vi "Load Default Measurements.vi"(8 "error in (no error)":errorcluster, 11 "Measurement Interface in":refnum<class "Measurement Interface.lvclass">) -> (0 "error out":errorcluster, 3 "Measurement Interface out":refnum<class "Measurement Interface.lvclass">)   [LabVIEW 2016, in "Measurement Interface.lvlib" / "Measurement Interface.lvclass"]
uses:
  Measurement Interface.lvclass
  Measurement Interface.lvclass/Measurement Interface.ctl
  Plugins/TestStand API Tools (TSAT).lvlibp/Sequence File Actions/TSAT Sequence File Actions.lvlib
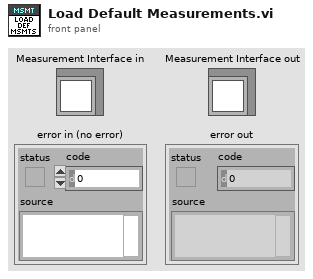
[diagram p1: front panel]
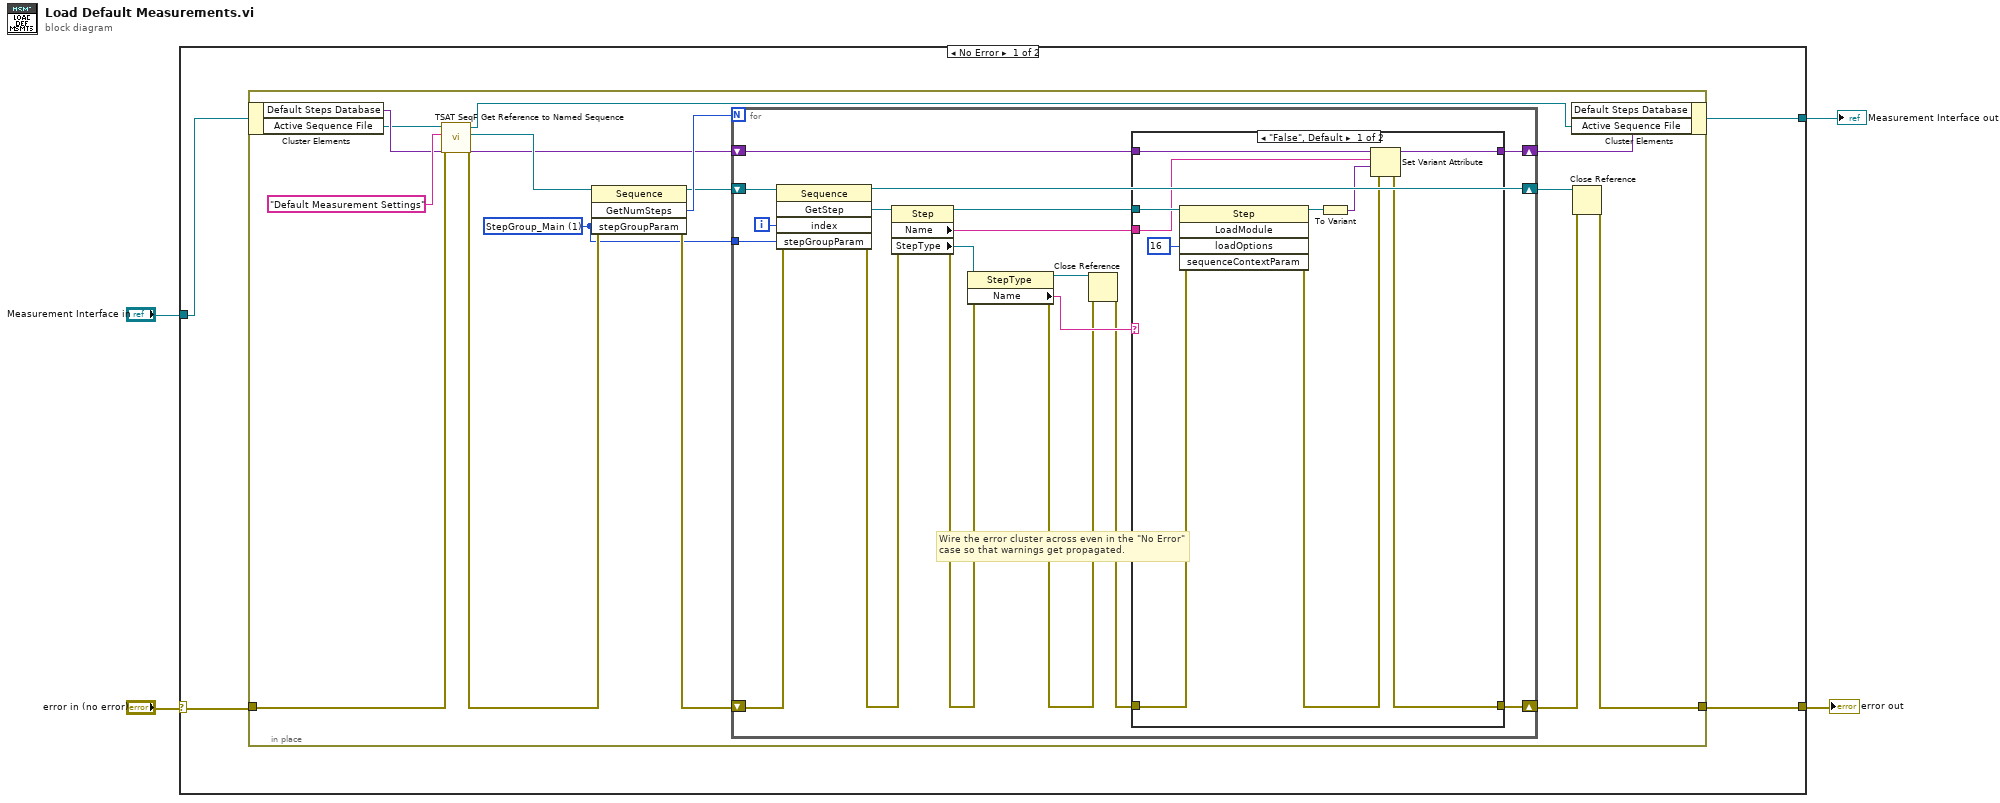
[diagram p0: block diagram]
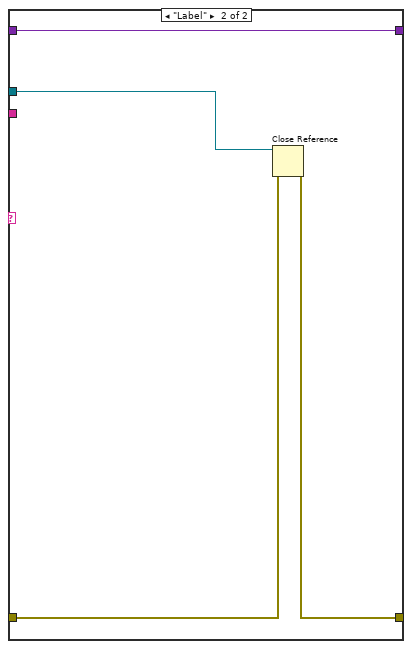
[diagram p2: hidden frame]
diagram:
  n1 = case shown="No Error" "error in (no error)" {
    selector: "error in (no error)" -> [w8 w57]
    tunnel: [w5 w57] -> w3
    tunnel: [w6 w56] -> w1
    tunnel: "Measurement Interface in" -> [w7 w56]
    frame No Error {
      # "Wire the error cluster across even in the \"No Error\"\ncase so that warnings get propagated."
      n2 = in-place {
        in-place-border: w8 -> [w23]
        in-place-border: [w11] -> w5
        w16 = 1 items=["StepGroup_Setup", "StepGroup_Main", "StepGroup_Cleanup"] ("stepGroupParam")
        n3 = in-place-cluster #1(w7) -> ("Default Steps Database"=w15:variant, "Active Sequence File"=w10:refnum<k7>)
        n4 = call "TSAT SeqF Get Reference to Named Sequence.vi"("Error In"=w23, "Seqeunce to Retrieve"="Default Measurement Settings", "Sequence File In"=w10) -> ("Error Out"=w20:errorcluster, "Named Sequence"=w21:refnum<k7>, "Sequence File Out"=w9:refnum<k7>)  [unwired: 6 in]
        n5 = invoke class="Sequence" method="GetNumSteps"(reference=w21, error in=w20, "stepGroupParam"=w16) -> (reference out=w18:refnum<k7>, error out=w17:errorcluster, "GetNumSteps"=w19:i32)  [unwired: 1 in, 1 out]
        n6 = for {
          N: w19 -> [_]
          shift-right: [w35] -> w13
          shift-left: w18 -> [w41]
          shift-right: [w29] -> w12
          shift-left: w17 -> [w39]
          tunnel: w16 -> [w38]
          shift-right: [w24] -> w14
          shift-left: w15 -> [w25]
          i -> [w40]
          n7 = invoke class="Sequence" method="GetStep"(reference=w41, error in=w39, "index"=w40, "stepGroupParam"=w38) -> (reference out=w35:refnum<k7>, error out=w36:errorcluster, "GetStep"=w37:refnum<k7>)  [unwired: 1 in, 2 out]
          n8 = property class="Step"(reference=w37, error in=w36) -> (reference out=w30:refnum<k7>, error out=w34:errorcluster, "Name"=w26:string, "StepType"=w27:refnum<k7>)
          n9 = property class="StepType"(reference=w27, error in=w34) -> (reference out=w32:refnum<k7>, error out=w31:errorcluster, "Name"=w33:string)
          n10 = Close Reference(reference=w32, error in (no error)=w31) -> (error out=w28:errorcluster)
          n11 = case shown="\"False\", Default" w33 {
            tunnel: w30 -> [w50 w55]
            tunnel: [w47 w53] -> w29
            tunnel: w28 -> [w44 w54]
            tunnel: w26 -> [w48 _]
            tunnel: w25 -> [w51 w52]
            tunnel: [w46 w52] -> w24
            frame "False", Default {
              n12 = invoke class="Step" method="LoadModule"(reference=w50, error in=w44, "loadOptions"=16) -> (reference out=w45:refnum<k7>, error out=w43:errorcluster)  [unwired: 2 in, 3 out]
              n13 = To Variant(anything=w45) -> (Variant=w49:variant)
              n14 = Set Variant Attribute(Variant=w51, name=w48, value=w49, error in=w43) -> (Variant out=w46:variant, error out=w47:errorcluster)  [unwired: 1 out]
            }
            frame "Label" {
              n15 = Close Reference(reference=w55, error in (no error)=w54) -> (error out=w53:errorcluster)
            }
          }
        }
        n16 = in-place-cluster #1("Default Steps Database"=w14, "Active Sequence File"=w9) -> (w6:refnum<class "Measurement Interface.lvclass">)
        n17 = Close Reference(reference=w13, error in (no error)=w12) -> (error out=w11:errorcluster)
      }
    }
    frame Error {
    }
  }
  "error out" <- w3
  "Measurement Interface out" <- w1
